vi "MGCC_Commun_tran_to_global.vi"() -> ()   [LabVIEW 2016]
uses:
  Global communication.vi
  Model Management (He Yin)/Global_MdlMgmt.vi
panel:
  in  "Empty array":dbl[](array[numeric])
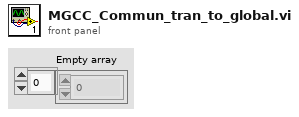
[diagram p1: front panel]
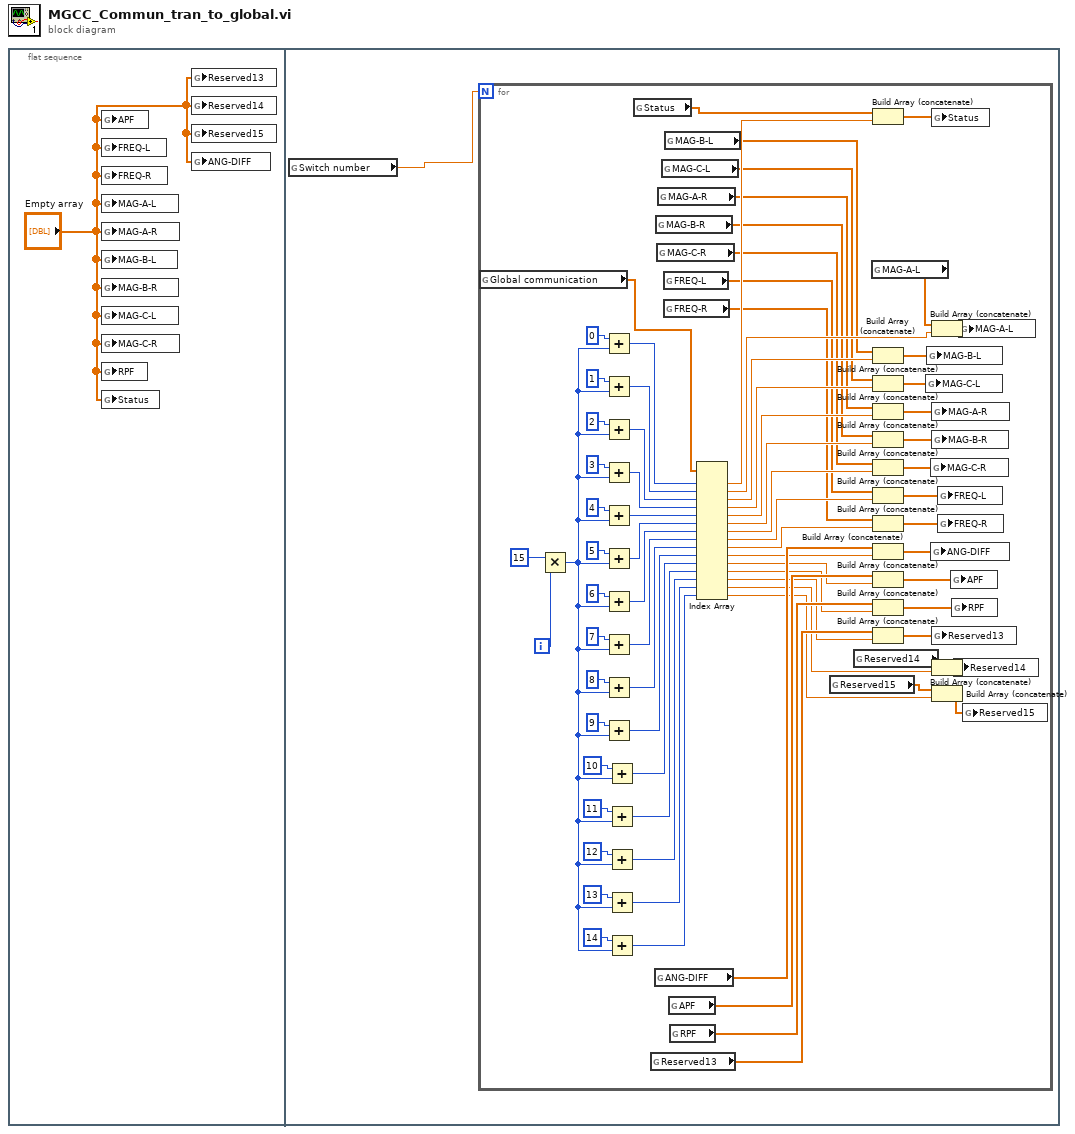
[diagram p0: block diagram]
diagram:
  n1 = flat-sequence {
    frame #0 {
      n2 = global write "Global communication.vi" "APF"("Empty array") -> ()
      n3 = global write "Global communication.vi" "FREQ-L"("Empty array") -> ()
      n4 = global write "Global communication.vi" "FREQ-R"("Empty array") -> ()
      n5 = global write "Global communication.vi" "MAG-A-L"("Empty array") -> ()
      n6 = global write "Global communication.vi" "MAG-A-R"("Empty array") -> ()
      n7 = global write "Global communication.vi" "MAG-B-L"("Empty array") -> ()
      n8 = global write "Global communication.vi" "MAG-B-R"("Empty array") -> ()
      n9 = global write "Global communication.vi" "MAG-C-L"("Empty array") -> ()
      n10 = global write "Global communication.vi" "MAG-C-R"("Empty array") -> ()
      n11 = global write "Global communication.vi" "RPF"("Empty array") -> ()
      n12 = global write "Global communication.vi" "Status"("Empty array") -> ()
      n13 = global write "Global communication.vi" "Reserved13"("Empty array") -> ()
      n14 = global write "Global communication.vi" "Reserved14"("Empty array") -> ()
      n15 = global write "Global communication.vi" "Reserved15"("Empty array") -> ()
      n16 = global write "Global communication.vi" "ANG-DIFF"("Empty array") -> ()
    }
    frame #1 {
      n17 = global read "Global_MdlMgmt.vi" "Switch number"() -> (w2:dbl)
      n18 = for {
        N: w2 -> [_]
        i -> [w11]
        n19 = global read "Global communication.vi" "Global communication"() -> (w9:dbl[])
        n20 = Multiply(x=15, y=w11) -> (x*y=w10:i32)
        n21 = Add(x=0 ("index"), y=w10) -> (x+y=w40:i32)
        n22 = Add(x=1 ("index"), y=w10) -> (x+y=w38:i32)
        n23 = Add(x=2 ("index"), y=w10) -> (x+y=w36:i32)
        n24 = Add(x=3 ("index"), y=w10) -> (x+y=w34:i32)
        n25 = Add(x=4 ("index"), y=w10) -> (x+y=w32:i32)
        n26 = Add(x=5 ("index"), y=w10) -> (x+y=w28:i32)
        n27 = Add(x=6 ("index"), y=w10) -> (x+y=w27:i32)
        n28 = Add(x=7 ("index"), y=w10) -> (x+y=w26:i32)
        n29 = Add(x=8 ("index"), y=w10) -> (x+y=w18:i32)
        n30 = Add(x=9 ("index"), y=w10) -> (x+y=w17:i32)
        n31 = Add(x=10 ("index"), y=w10) -> (x+y=w16:i32)
        n32 = Add(x=11 ("index"), y=w10) -> (x+y=w15:i32)
        n33 = Add(x=12 ("index"), y=w10) -> (x+y=w14:i32)
        n34 = Add(x=13 ("index"), y=w10) -> (x+y=w13:i32)
        n35 = Add(x=14 ("index"), y=w10) -> (x+y=w12:i32)
        n36 = global read "Global communication.vi" "Status"() -> (w7:dbl[])
        n37 = global read "Global communication.vi" "Reserved13"() -> (w48:dbl[])
        n38 = global read "Global communication.vi" "ANG-DIFF"() -> (w57:dbl[])
        n39 = global read "Global communication.vi" "MAG-B-R"() -> (w68:dbl[])
        n40 = global read "Global communication.vi" "MAG-C-R"() -> (w65:dbl[])
        n41 = global read "Global communication.vi" "MAG-A-R"() -> (w71:dbl[])
        n42 = global read "Global communication.vi" "MAG-C-L"() -> (w74:dbl[])
        n43 = global read "Global communication.vi" "FREQ-L"() -> (w3:dbl[])
        n44 = global read "Global communication.vi" "FREQ-R"() -> (w60:dbl[])
        n45 = global read "Global communication.vi" "MAG-B-L"() -> (w77:dbl[])
        n46 = global read "Global communication.vi" "APF"() -> (w54:dbl[])
        n47 = global read "Global communication.vi" "RPF"() -> (w51:dbl[])
        n48 = Index Array(array=w9, index #1=w40, index #2=w38, index #3=w36, index #4=w34, index #5=w32, index #6=w28, index #7=w27, index #8=w26, index #9=w18, index #10=w17, index #11=w16, index #12=w15, index #13=w14, index #14=w13, index #15=w12) -> (element #1=w81:dbl, element #2=w79:dbl, element #3=w76:dbl, element #4=w73:dbl, element #5=w70:dbl, element #6=w67:dbl, element #7=w64:dbl, element #8=w62:dbl, element #9=w59:dbl, element #10=w56:dbl, element #11=w53:dbl, element #12=w50:dbl, element #13=w47:dbl, element #14=w43:dbl, element #15=w42:dbl)
        n49 = global read "Global communication.vi" "Reserved15"() -> (w5:dbl[])
        n50 = global read "Global communication.vi" "Reserved14"() -> (w45:dbl[])
        n51 = global read "Global communication.vi" "MAG-A-L"() -> (w80:dbl[])
        n52 = Build Array (concatenate)(w7, w81) -> (w6:dbl[])
        n53 = Build Array (concatenate)(w77, w76) -> (w75:dbl[])
        n54 = Build Array (concatenate)(w74, w73) -> (w72:dbl[])
        n55 = Build Array (concatenate)(w71, w70) -> (w69:dbl[])
        n56 = Build Array (concatenate)(w68, w67) -> (w66:dbl[])
        n57 = Build Array (concatenate)(w65, w64) -> (w63:dbl[])
        n58 = Build Array (concatenate)(w3, w62) -> (w61:dbl[])
        n59 = Build Array (concatenate)(w60, w59) -> (w58:dbl[])
        n60 = Build Array (concatenate)(w57, w56) -> (w55:dbl[])
        n61 = Build Array (concatenate)(w54, w53) -> (w52:dbl[])
        n62 = Build Array (concatenate)(w51, w50) -> (w49:dbl[])
        n63 = Build Array (concatenate)(w48, w47) -> (w46:dbl[])
        n64 = global write "Global communication.vi" "MAG-C-L"(w72) -> ()
        n65 = global write "Global communication.vi" "MAG-B-L"(w75) -> ()
        n66 = global write "Global communication.vi" "MAG-C-R"(w63) -> ()
        n67 = global write "Global communication.vi" "ANG-DIFF"(w55) -> ()
        n68 = global write "Global communication.vi" "Status"(w6) -> ()
        n69 = Build Array (concatenate)(w80, w79) -> (w78:dbl[])
        n70 = global write "Global communication.vi" "MAG-A-R"(w69) -> ()
        n71 = global write "Global communication.vi" "MAG-B-R"(w66) -> ()
        n72 = global write "Global communication.vi" "Reserved13"(w46) -> ()
        n73 = Build Array (concatenate)(w45, w43) -> (w44:dbl[])
        n74 = Build Array (concatenate)(w5, w42) -> (w4:dbl[])
        n75 = global write "Global communication.vi" "FREQ-L"(w61) -> ()
        n76 = global write "Global communication.vi" "FREQ-R"(w58) -> ()
        n77 = global write "Global communication.vi" "APF"(w52) -> ()
        n78 = global write "Global communication.vi" "RPF"(w49) -> ()
        n79 = global write "Global communication.vi" "Reserved14"(w44) -> ()
        n80 = global write "Global communication.vi" "MAG-A-L"(w78) -> ()
        n81 = global write "Global communication.vi" "Reserved15"(w4) -> ()
      }
    }
  }
